vi "Add Lockin Comments.vi"(7 "error in (no error)":errorcluster, 9 "Channels: AO":T1={"AO amp (V)"=[0.01, 0.0, 0.0, 0.0, 0.0, 0.0, 0.0, 0.0], "AO DC (V)"=[0.0, 0.0, 0.0, 0.0, 0.0, 0.0, 0.0, 0.0], "AO f (Hz)"=[13.1, 13.0, 13.0, 13.0, 13.0, 13.0, 13.0, 13.0], "AO phi (°)"=[0.0, 0.0, 0.0, 0.0, 0.0, 0.0, 0.0, 0.0], "function"=[], "I+"=[]} {"AO f (Hz)" min=0.001 max=10000.0; "AO DC (V)" format="%.3p"; "AO amp (V)" format="%.3p"}, 10 "Comments in":string) -> (0 "error out":errorcluster, 3 "Comments":string)   [LabVIEW 2016, in "Control Experiment.lvclass"]
uses:
  Control Experiment.lvclass
  <userlib>/LevyLab/Lockin-Multichannel/Typedefs/AO-cluster.ctl
  <userlib>/LevyLab/Lockin-Multichannel/Typedefs/AO_Amp-array.ctl
  <userlib>/LevyLab/Lockin-Multichannel/Typedefs/AO_DC-array.ctl
  <userlib>/LevyLab/Lockin-Multichannel/Typedefs/AO_f-array.ctl
  <userlib>/LevyLab/Lockin-Multichannel/Typedefs/AO_phi-array.ctl
  <userlib>/LevyLab/Lockin-Multichannel/Typedefs/Function-array.ctl
  <userlib>/LevyLab/Lockin-Multichannel/Typedefs/Function-enum.ctl
panel:
  # "1"
  # "2"
  # "3"
  # "4"
  # "5"
  # "6"
  # "7"
  # "8"
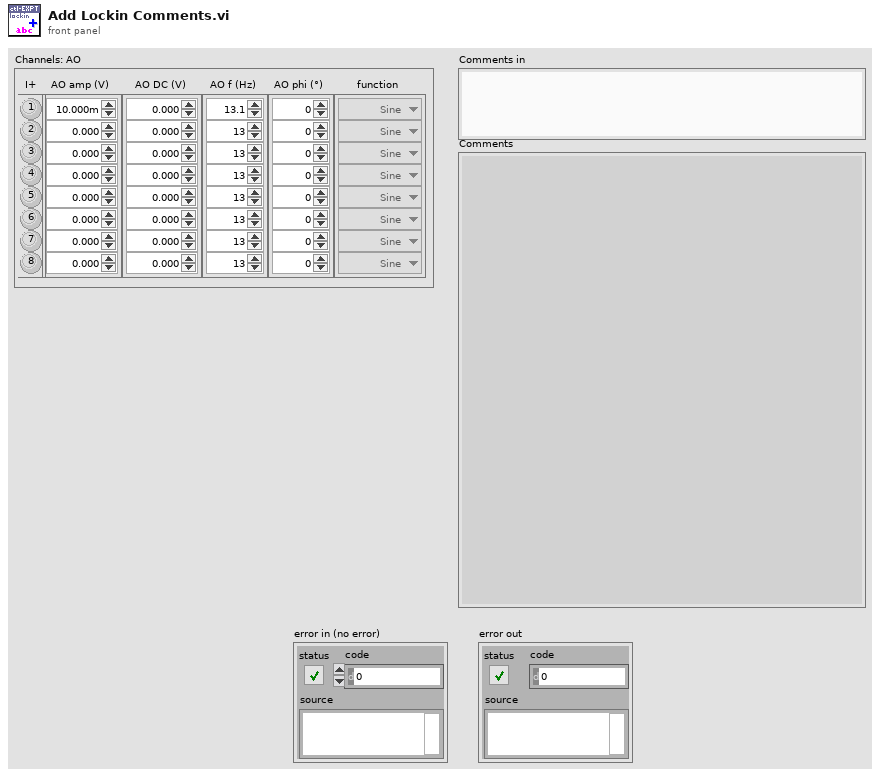
[diagram p1: front panel]
types:
  T1 = typedef "AO-cluster.ctl" = cluster{"AO amp (V)":T2, "AO DC (V)":T3, "AO f (Hz)":T4, "AO phi (°)":T5, "function":T6, "I+":bool[]}
  T2 = typedef "AO_Amp-array.ctl" = dbl[]
  T3 = typedef "AO_DC-array.ctl" = dbl[]
  T4 = typedef "AO_f-array.ctl" = dbl[]
  T5 = typedef "AO_phi-array.ctl" = dbl[]
  T6 = typedef "Function-array.ctl" = T7[]
  T7 = typedef "Function-enum.ctl" = enum16{"Sine", "Triangle", "Square", "Sawtooth"}
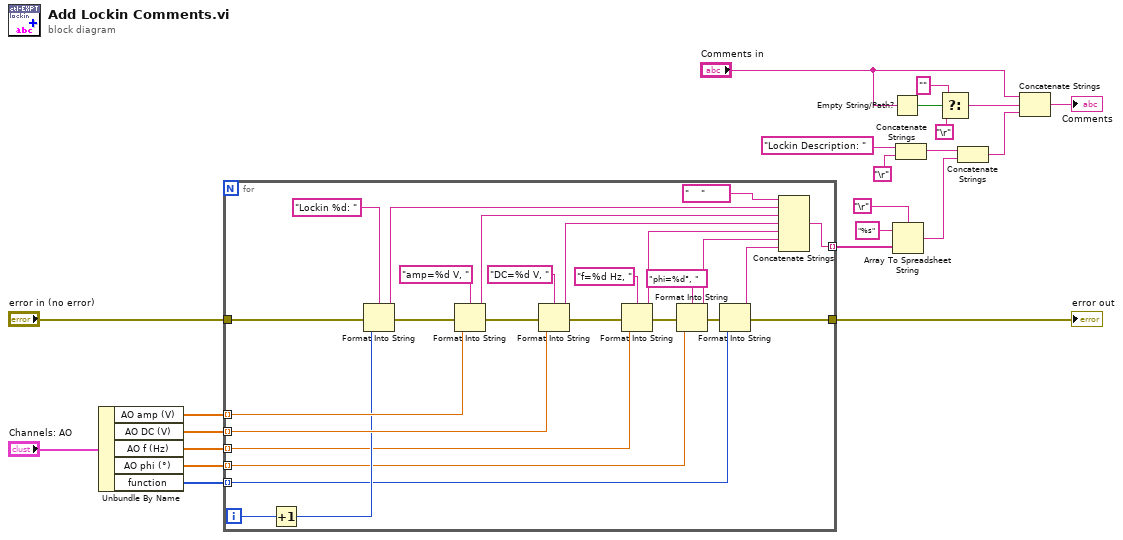
[diagram p0: block diagram]
diagram:
  n1 = Unbundle By Name("Channels: AO") -> ("AO amp (V)"=w18:T2, "AO DC (V)"=w19:T3, "AO f (Hz)"=w20:T4, "AO phi (°)"=w21:T5, "function"=w22:T6)
  n2 = for {
    tunnel: w18 -> [w34] mode=indexing
    tunnel: w19 -> [w35] mode=indexing
    tunnel: w20 -> [w30] mode=indexing
    tunnel: w21 -> [w28] mode=indexing
    tunnel: w22 -> [w29] mode=indexing
    tunnel: [w49] -> w13 mode=indexing
    tunnel: "error in (no error)" -> [w48]
    tunnel: [w43] -> w12
    i -> [w41]
    n3 = Increment(x=w41) -> (x+1=w33:i32)
    n4 = Format Into String(format string="Lockin %d: ", error in=w48, w33) -> (resulting string=w38:string, error out=w47:errorcluster)  [unwired: 1 in]
    n5 = Format Into String(format string="amp=%d V, ", error in=w47, w34) -> (resulting string=w37:string, error out=w42:errorcluster)  [unwired: 1 in]
    n6 = Format Into String(format string="DC=%d V, ", error in=w42, w35) -> (resulting string=w32:string, error out=w46:errorcluster)  [unwired: 1 in]
    n7 = Format Into String(format string="f=%d Hz, ", error in=w46, w30) -> (resulting string=w27:string, error out=w45:errorcluster)  [unwired: 1 in]
    n8 = Format Into String(format string="phi=%d°, ", error in=w45, w28) -> (resulting string=w25:string, error out=w44:errorcluster)  [unwired: 1 in]
    n9 = Format Into String(error in=w44, w29) -> (resulting string=w24:string, error out=w43:errorcluster)  [unwired: 2 in]
    n10 = Concatenate Strings("    " ("string"), w38, w37, w32, w27, w25, w24) -> (w49:string)
  }
  "error out" <- w12
  n11 = Empty String/Path?(string/path="Comments in") -> (empty?=w5:bool)
  n12 = Array To Spreadsheet String(delimiter (Tab)="\r", array=w13, 3:"%s" ("format string")) -> (spreadsheet string=w8:string)
  n13 = Concatenate Strings("Lockin Description: " ("string"), "\r") -> (w9:string)
  n14 = Select(t="", s=w5, f="\r") -> (s? t:f=w2:string)
  n15 = Concatenate Strings(w9, w8) -> (w7:string)
  n16 = Concatenate Strings("Comments in", w2, w7) -> (→"Comments":string)
